vi "Teleop.vi"(10 "Match Info":T1={"Autonomous Elapsed Seconds"=0.0, "TeleOp Elapsed Seconds"=0.0, "Disabled Elapsed Seconds"=0.0, "Visited Autonomous"=FALSE, "Visited TeleOp"=FALSE, "Visited Disabled"=FALSE, "Autonomous Settings"={"Autonomous Style"=enum."Independent", "VI Refnum"=refnum}}, 11 "Call Context":T2) -> ()   [LabVIEW 2023]
doc: "This VI is called for each TeleOp packet received from the DS where the robot is not disabled. It is often used to read from the joysticks and update I/O or to update setpoints for timed control loops. It should complete and return within 20 milliseconds or it may miss DS packets."
uses:
  <vilib>/Rock Robotics/WPI/DriverStation/WPI_DriverStationDerivedRobotMode.ctl
  <vilib>/Rock Robotics/WPI/DriverStation/WPI_DriverStationMatch Info.ctl
  <vilib>/Rock Robotics/Network Tables/NT Read Boolean.vi
  <vilib>/Rock Robotics/Network Tables/NT Read Number.vi
  <vilib>/Rock Robotics/WPI/Utilities/WPI_GetSetVariantRefNum.vi
  Robot Global Data.vi
  <vilib>/addons/control/pid/pid.llb/PID Output Rate Limiter (DBL).vi
  <vilib>/addons/control/pid/NI_PID_pid.lvlib
panel:
  out "Sample Slider 0":dbl(slide) scale=0.0..5.0
  out "Sample Boolean 1":bool
  out "Sample Boolean 0":bool
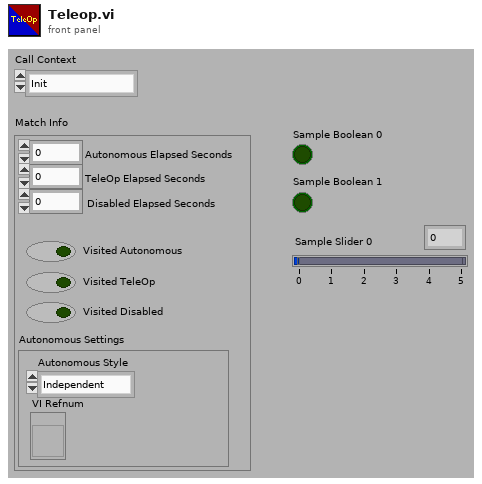
[diagram p1: front panel]
types:
  T1 = typedef "WPI_DriverStationMatch Info.ctl" = cluster{"Autonomous Elapsed Seconds":dbl, "TeleOp Elapsed Seconds":dbl, "Disabled Elapsed Seconds":dbl, "Visited Autonomous":bool, "Visited TeleOp":bool, "Visited Disabled":bool, "Autonomous Settings":cluster{"Autonomous Style":enum16{"Iterative", "Independent"}, "VI Refnum":refnum<vi>}}
  T2 = typedef "WPI_DriverStationDerivedRobotMode.ctl" = enum16{"Init", "Execute", "Stop"}
  T3 = typedef "WPI_JoystickDevRef.ctl" = cluster{"Device":T4}
  T4 = typedef "WPI_JoystickDeviceEnum.ctl" = enum16{"USB 0", "USB 1", "USB 2", "USB 3", "USB 4", "USB 5"}
  T5 = typedef "WPI_RobotDriveDevRef.ctl" = cluster{"DevStatus":errorcluster, "Motors[]":T6[], "Square Inputs":bool, "Max Output":dbl}
  T6 = typedef "WPI_MotorControlDeviceRef.ctl" = cluster{"DeviceStatus":errorcluster, "Type":T7, "PWM":cluster{"PWM Channel":T8, "DeadBand":T9}, "CAN":cluster{"Device Number":u8, "SetOutput VI Ref":variant, "GetOutput VI Ref":variant, "Enable VI Ref":variant, "Disable VI Ref":variant, "Data":variant}, "Invert":bool, "DIO PWM":cluster{"PWM \"Enable\" Channel":T8, "DIOChannel":T10, "PWM Rate":dbl}}
  T7 = typedef "WPI_MotorControlType.ctl" = enum16{"PWM", "CAN", "DIO PWM"}
  T8 = typedef "FPGA_DIOPWMChannel.ctl" = enum8{"PWM 0", "PWM 1", "PWM 2", "PWM 3", "PWM 4", "PWM 5", "PWM 6", "PWM 7", "PWM 8", "PWM 9", "PWM MXP 0", "PWM MXP 1", "PWM MXP 2", "PWM MXP 3", "PWM MXP 4", "PWM MXP 5", "PWM MXP 6", "PWM MXP 7", "PWM MXP 8", "PWM MXP 9", "Invalid"}
  T9 = typedef "WPI_PWMDeadband.ctl" = cluster{"Name":string, "maxPositivePwm":i32, "minPositivePwm":i32, "centerPwm":i32, "maxNegativePwm":i32, "minNegativePwm":i32, "angularRange":u16}
  T10 = typedef "FPGA_DIOChannel.ctl" = enum8{"DIO 0", "DIO 1", "DIO 2", "DIO 3", "DIO 4", "DIO 5", "DIO 6", "DIO 7", "DIO 8", "DIO 9", "DIO MXP 0", "DIO MXP 1", "DIO MXP 2", "DIO MXP 3", "DIO MXP 4", "DIO MXP 5", "DIO MXP 6", "DIO MXP 7", "DIO MXP 8", "DIO MXP 9", "DIO MXP 10", "DIO MXP 11", "DIO MXP 12", "DIO MXP 13", "DIO MXP 14", "DIO MXP 15", "SPI Port CS1", "SPI Port CS2", "SPI Port CS3", "SPI Port MISO", "SPI Port MOSI", "Invalid"}
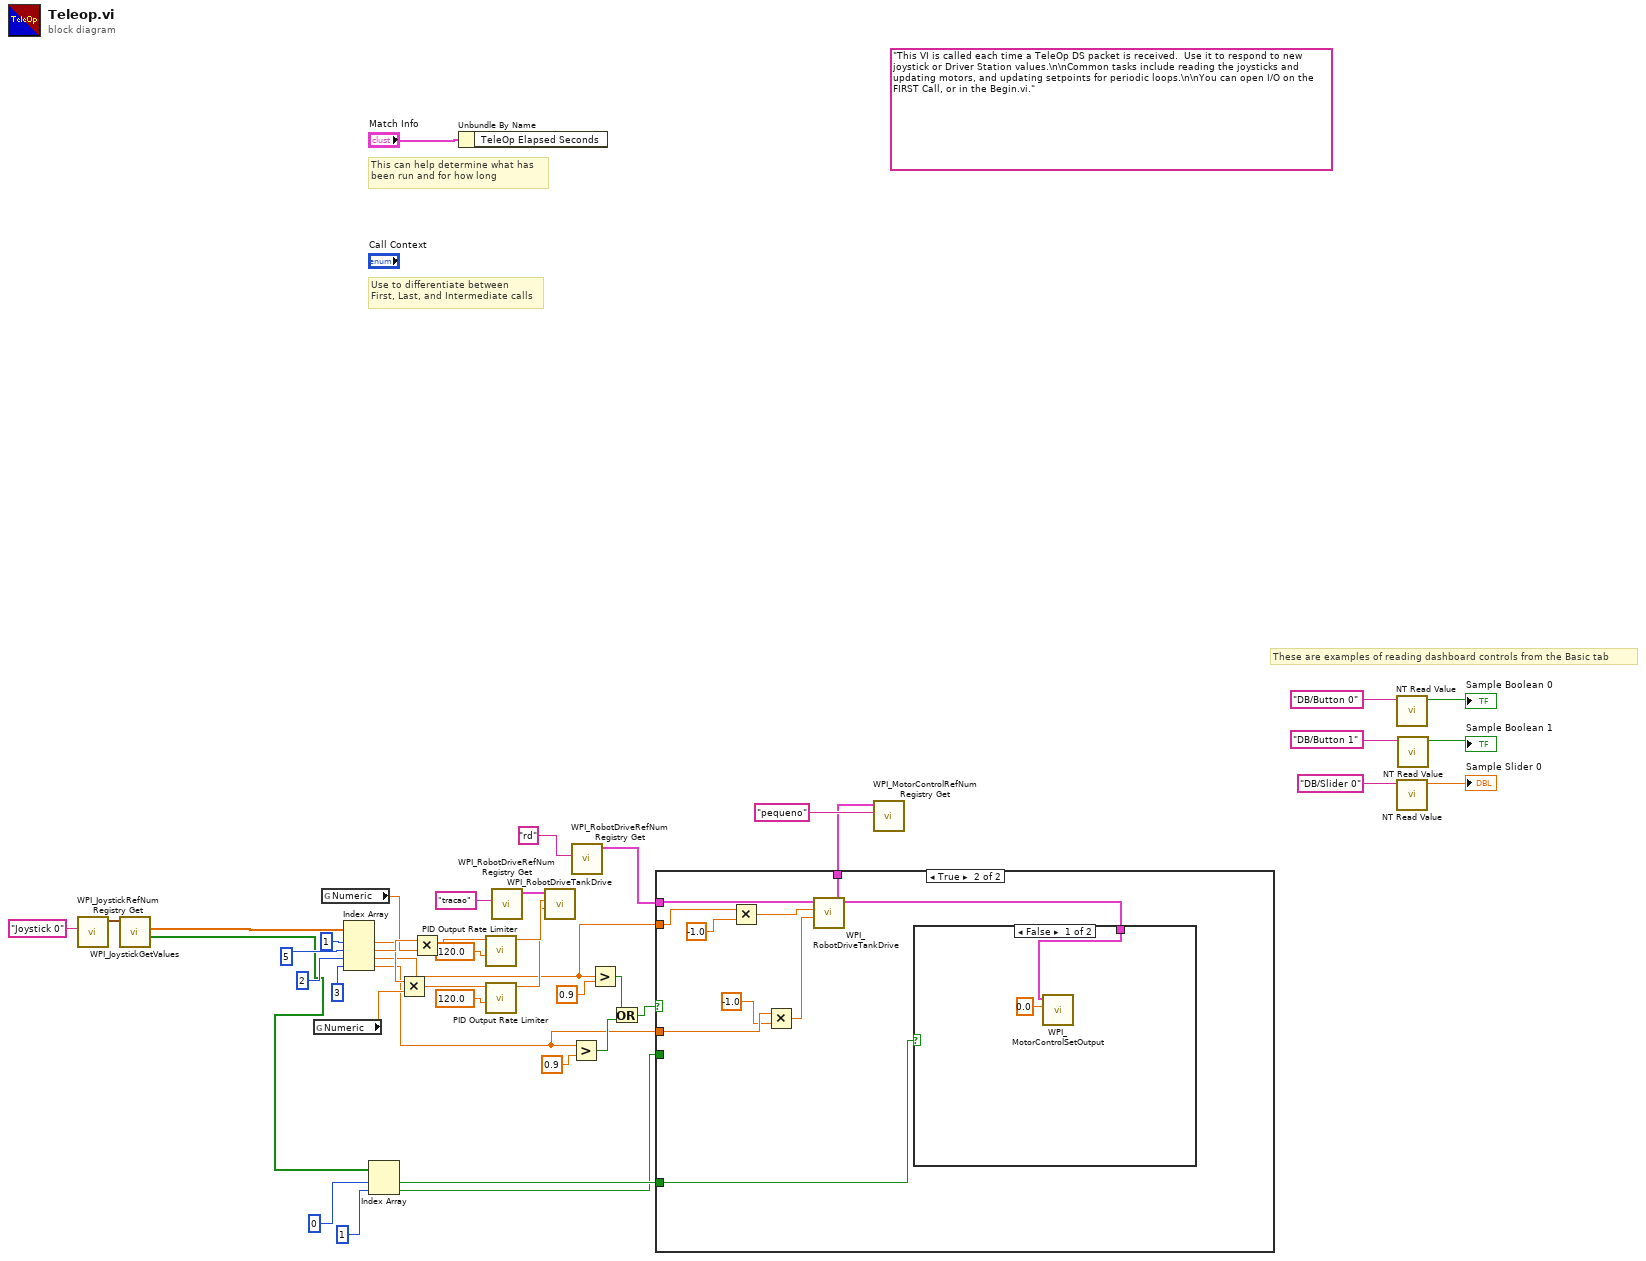
[diagram p0: block diagram]
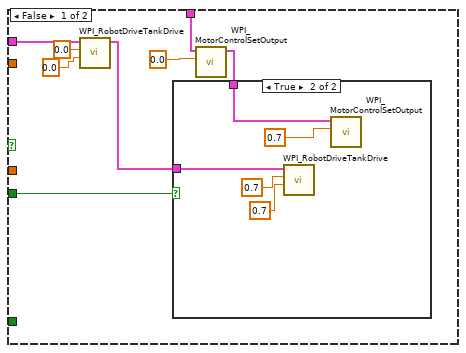
[diagram p2: hidden frame]
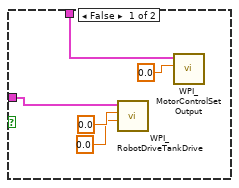
[diagram p3: hidden frame]
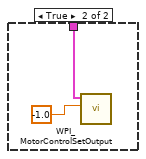
[diagram p4: hidden frame]
diagram:
  (unwired) "This VI is called each time a TeleOp DS packet is received.  Use it to respond to new joystick or Driver Station values.\n\nCommon tasks include reading the joysticks and updating motors, and updating setpoints for periodic loops.\n\nYou can open I/O on the FIRST Call, or in the Begin.vi."
  # "These are examples of reading dashboard controls from the Basic tab"
  # "Use to differentiate between\nFirst, Last, and Intermediate calls"
  # "This can help determine what has\nbeen run and for how long"
  n1 = call <vilib>:"WPI_JoystickRefNum Registry Get.vi"("refnum name"="Joystick 0") -> ("JoystickDevRef"=w34:T3)  [unwired: 9 in, 1 out]
  n2 = call <vilib>:"WPI_JoystickGetValues.vi"("JoystickDevRef"=w34) -> ("Buttons"=w6:bool[], "Axes"=w30:dbl[])  [unwired: 6 in, 3 out]
  n3 = global read "Robot Global Data.vi" "Numeric"() -> (w20:dbl)
  n4 = global read "Robot Global Data.vi" "Numeric"() -> (w19:dbl)
  n5 = Index Array(array=w30, index #1=1 ("index"), index #2=5 ("index"), index #3=2 ("index"), index #4=3 ("index")) -> (element #1=w24:dbl, element #2=w26:dbl, element #3=w9:dbl, element #4=w8:dbl)
  n6 = Index Array(array=w6, index #1=0 ("index"), index #2=1 ("index")) -> (element #1=w5:bool, element #2=w1:bool)
  n7 = Multiply(x=w24, y=w20) -> (x*y=w23:dbl)
  n8 = Multiply(x=w26, y=w19) -> (x*y=w25:dbl)
  n9 = Unbundle By Name("Match Info") -> ()  [unwired: 1 out]
  n10 = call-poly <vilib>:"PID Output Rate Limiter.vi"("output rate (EGU/min)"=120.0 ("output rate (EGU/min) 2"), "input (controller output)"=w25) -> ("output"=w22:dbl)  [unwired: 6 in, 1 out]
  n11 = call-poly <vilib>:"PID Output Rate Limiter.vi"("output rate (EGU/min)"=120.0, "input (controller output)"=w23) -> ("output"=w21:dbl)  [unwired: 6 in, 1 out]
  n12 = call <vilib>:"WPI_RobotDriveRefNum Registry Get.vi"("refnum name"="tracao") -> ("RobotDriveDevRef"=w27:T5)  [unwired: 9 in, 1 out]
  n13 = call <vilib>:"WPI_RobotDriveTankDrive.vi"("Right axis value"=w21, "Left axis value"=w22, "RobotDriveDevRef"=w27) -> ()  [unwired: 6 in, 3 out]
  n14 = Greater?(x=w8, y=0.9) -> (0:w13:bool)
  n15 = call <vilib>:"WPI_RobotDriveRefNum Registry Get.vi"("refnum name"="rd") -> ("RobotDriveDevRef"=w10:T5)  [unwired: 9 in, 1 out]
  n16 = Greater?(x=w9, y=0.9) -> (0:w14:bool)
  n17 = Or(x=w14, y=w13) -> (x .or. y?=w12:bool)
  n18 = call <vilib>:"WPI_MotorControlRefNum Registry Get.vi"("refnum name"="pequeno") -> ("MotorControlDevRef"=w3:T6)  [unwired: 9 in, 1 out]
  n19 = case shown="True" w12 {
    tunnel: w10 -> [w50 w69]
    tunnel: w9 -> [_ w65]
    tunnel: w8 -> [_ w66]
    tunnel: w5 -> [_ w67]
    tunnel: w3 -> [w46 w68]
    tunnel: w1 -> [w45 _]
    frame False {
      n20 = call <vilib>:"WPI_RobotDriveTankDrive.vi"("Right axis value"=0.0 ("Left axis value"), "Left axis value"=0.0, "RobotDriveDevRef"=w50) -> ("RobotDriveDevRef"=w44:T5)  [unwired: 6 in, 2 out]
      n21 = call <vilib>:"WPI_MotorControlSetOutput.vi"("Output"=0.0, "MotorControlDevRef"=w46) -> ("MotorControlDevRef"=w43:T6)  [unwired: 7 in, 2 out]
      n22 = case shown="True" w45 {
        tunnel: w44 -> [w55 w60]
        tunnel: w43 -> [w52 w57]
        frame False {
          n23 = call <vilib>:"WPI_RobotDriveTankDrive.vi"("Right axis value"=0.0 ("Left axis value"), "Left axis value"=0.0, "RobotDriveDevRef"=w55) -> ()  [unwired: 6 in, 3 out]
          n24 = call <vilib>:"WPI_MotorControlSetOutput.vi"("Output"=0.0, "MotorControlDevRef"=w52) -> ()  [unwired: 7 in, 3 out]
        }
        frame True {
          n25 = call <vilib>:"WPI_RobotDriveTankDrive.vi"("Right axis value"=0.7, "Left axis value"=0.7, "RobotDriveDevRef"=w60) -> ()  [unwired: 6 in, 3 out]
          n26 = call <vilib>:"WPI_MotorControlSetOutput.vi"("Output"=0.7, "MotorControlDevRef"=w57) -> ()  [unwired: 7 in, 3 out]
        }
      }
    }
    frame True {
      n27 = Multiply(x=w65, y=-1.0) -> (x*y=w62:dbl)
      n28 = Multiply(x=w66, y=-1.0) -> (x*y=w61:dbl)
      n29 = call <vilib>:"WPI_RobotDriveTankDrive.vi"("Right axis value"=w61, "Left axis value"=w62, "RobotDriveDevRef"=w69) -> ()  [unwired: 6 in, 3 out]
      n30 = case shown="False" w67 {
        tunnel: w68 -> [w71 w73]
        frame False {
          n31 = call <vilib>:"WPI_MotorControlSetOutput.vi"("Output"=0.0, "MotorControlDevRef"=w71) -> ()  [unwired: 7 in, 3 out]
        }
        frame True {
          n32 = call <vilib>:"WPI_MotorControlSetOutput.vi"("Output"=-1.0, "MotorControlDevRef"=w73) -> ()  [unwired: 7 in, 3 out]
        }
      }
    }
  }
  n33 = call-poly <vilib>:"NT Read Value.vi"("name"="DB/Button 0" ("refnum name")) -> ("value"=→"Sample Boolean 0":bool)  [unwired: 8 in, 2 out]
  n34 = call-poly <vilib>:"NT Read Value.vi"("name"="DB/Slider 0" ("refnum name")) -> ("value"=→"Sample Slider 0":dbl)  [unwired: 8 in, 2 out]
  n35 = call-poly <vilib>:"NT Read Value.vi"("name"="DB/Button 1" ("refnum name")) -> ("value"=→"Sample Boolean 1":bool)  [unwired: 8 in, 2 out]
